vi "Get Control Information.vi"(8 "error in (no error)":errorcluster, 11 "Table in":refnum<class "Table.lvclass">) -> (0 "error out":errorcluster, 2 "Control Information":string[][](array[string]), 3 "Table out":refnum<class "Table.lvclass">)   [LabVIEW 2017, in "Localization.lvlib" / "Table.lvclass"]
doc: "VI for override that is supposed to do go throgh the process for each control type and pull out the information that is necessary for each control.\n\nChoose Movement Consulting, LLC"
uses:
  Table.lvclass
  C:/Apps/CMC/OpenSource/Localization/Control Info/Control Info.lvclass
  Localization.lvlib
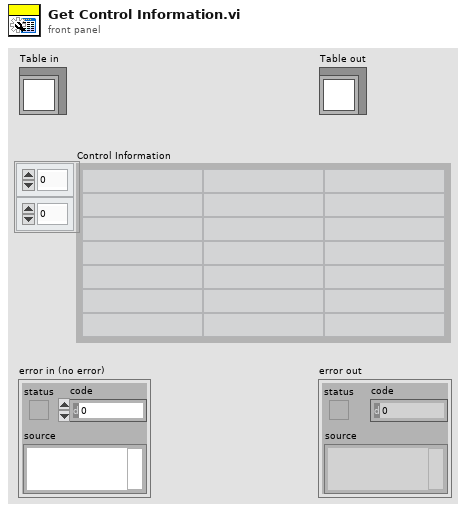
[diagram p1: front panel]
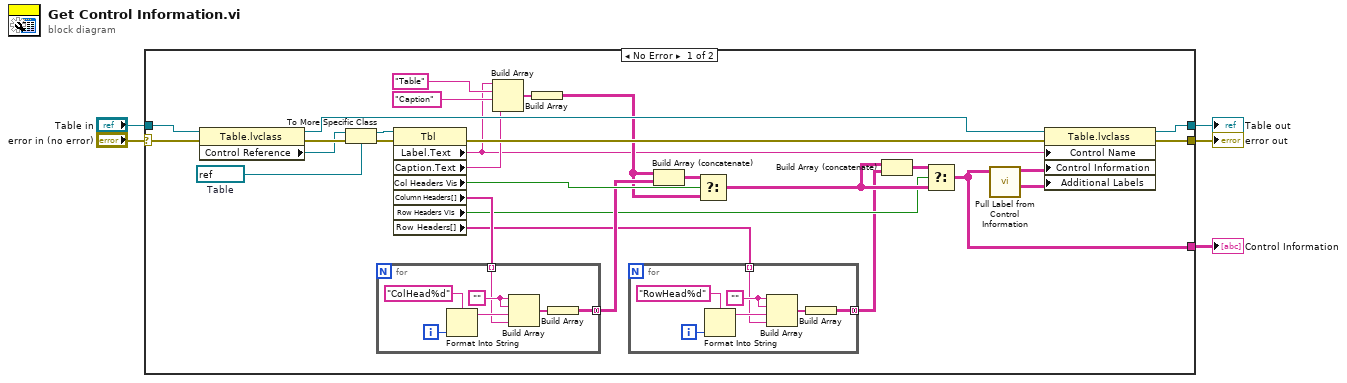
[diagram p0: block diagram]
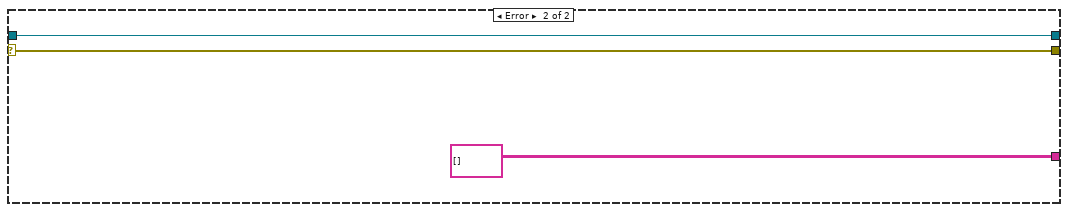
[diagram p2: hidden frame]
diagram:
  n1 = case shown="No Error" "error in (no error)" {
    selector: "error in (no error)" -> [w29 w51]
    tunnel: [w25 w51] -> w4
    tunnel: "Table in" -> [w28 w50]
    tunnel: [w9 string[][] []] -> w3
    tunnel: [w23 w50] -> w2
    frame No Error {
      w34 = refnum<vi> refnum  # Table
      n2 = property class="Table.lvclass"(reference=w28, error in=w29) -> (reference out=w24:refnum<class "Table.lvclass">, error out=w30:errorcluster, "Control Reference"=w27:refnum<vi>)
      n3 = To More Specific Class(target class=w34, reference=w27, error in=w30) -> (specific class reference=w33:refnum<vi>, error out=w31:errorcluster)
      n4 = property class="Tbl"(reference=w33, error in=w31) -> (error out=w26:errorcluster, "Label.Text"=w6:string, "Caption.Text"=w10:string, "Col Headers Vis"=w22:bool, "Column Headers[]"=w21:string[], "Row Headers Vis"=w13:bool, "Row Headers[]"=w12:string[])  [unwired: 1 out]
      n5 = for {
        tunnel: w21 -> [w42] mode=indexing
        tunnel: [w47] -> w20 mode=concatenating
        i -> [w44]
        w46 = ""
        n6 = Format Into String(format string="ColHead%d", w44) -> (resulting string=w43:string)  [unwired: 2 in, 1 out]
        n7 = Build Array(w46, w46, w43, w42) -> (w48:string[])
        n8 = Build Array(w48) -> (w47:string[][])
      }
      n9 = Build Array(w6, "Table", "Caption", w10) -> (w32:string[])
      n10 = Build Array(w32) -> (w19:string[][])
      n11 = for {
        tunnel: w12 -> [w35] mode=indexing
        tunnel: [w40] -> w11 mode=concatenating
        i -> [w37]
        w39 = ""
        n12 = Format Into String(format string="RowHead%d", w37) -> (resulting string=w36:string)  [unwired: 2 in, 1 out]
        n13 = Build Array(w39, w39, w36, w35) -> (w41:string[])
        n14 = Build Array(w41) -> (w40:string[][])
      }
      n15 = Build Array (concatenate)(w19, w20) -> (w18:string[][])
      n16 = Select(t=w18, s=w22, f=w19) -> (s? t:f=w14:string[][])
      n17 = Build Array (concatenate)(w14, w11) -> (w15:string[][])
      n18 = Select(t=w15, s=w13, f=w14) -> (s? t:f=w9:string[][])
      n19 = call "Pull Label from Control Information.vi"("Control Caption Table"=w9) -> ("Additional Labels"=w7:string[][], "Control Information"=w8:string[][])  [unwired: 9 in]
      n20 = property class="Table.lvclass"(reference=w24, error in=w26, "Control Name"=w6, "Control Information"=w8, "Additional Labels"=w7) -> (reference out=w23:refnum<class "Table.lvclass">, error out=w25:errorcluster)
    }
    frame Error {
    }
  }
  "error out" <- w4
  "Table out" <- w2
  "Control Information" <- w3
